vi "Get SubroutineInfo.vi"(11 "error in (no error)":errorcluster) -> (4 "data":T1, 15 "error out":errorcluster)   [LabVIEW 2021, in "Migrator Reusables.lvlib"]
uses:
  Migrator Reusables.lvlib
  controls/ErrorInformation.ctl
  controls/Dictionary States.ctl
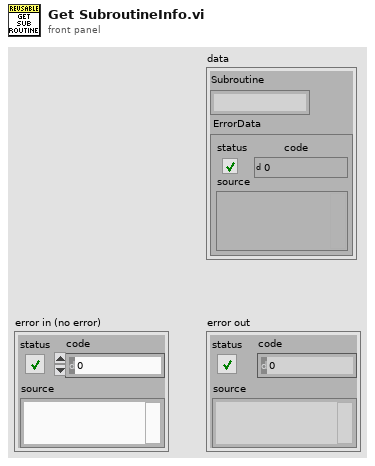
[diagram p1: front panel]
types:
  T1 = typedef "Migrator Reusables.lvlib/ErrorInformation.ctl" = cluster{"Subroutine":string, "ErrorData":errorcluster}
  T2 = typedef "Migrator Reusables.lvlib/Dictionary States.ctl" = enum16{"Set", "Get", "Delete", "Delete All"}
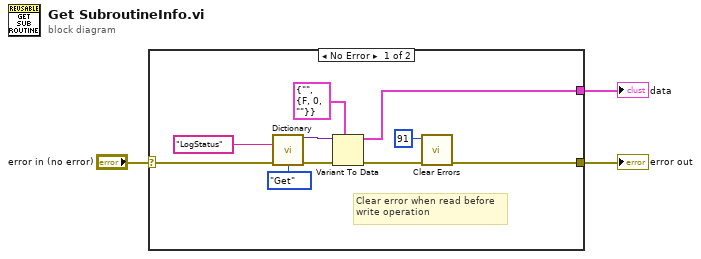
[diagram p0: block diagram]
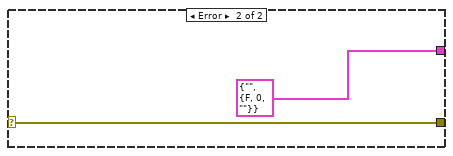
[diagram p2: hidden frame]
diagram:
  n1 = case shown="No Error" "error in (no error)" {
    selector: "error in (no error)" -> [w13 w15]
    tunnel: [w4 w15] -> w2
    tunnel: [w7 T1 {"Subroutine"="", "ErrorData"={"status"=FALSE, "code"=0, "source"=""}} ("ErrorInformation")] -> w1
    frame No Error {
      # "Clear error when read before\nwrite operation"
      n2 = call "Dictionary.vi"("Key"="LogStatus", "error in (no error)"=w13, "Dict States"=Dictionary_States."Get") -> ("Variant_Out"=w11:variant, "error out"=w12:errorcluster)  [unwired: 11 in]
      n3 = Variant To Data(error in=w12, type=T1 {"Subroutine"="", "ErrorData"={"status"=FALSE, "code"=0, "source"=""}} ("ErrorInformation"), Variant=w11) -> (data=w7:T1, error out=w6:errorcluster)
      n4 = call <vilib>:"Clear Errors.vi"("error in (no error)"=w6, "specific error code to clear (0: all)"=91) -> ("error out"=w4:errorcluster)  [unwired: 4 in, 1 out]
    }
    frame Error {
    }
  }
  "error out" <- w2
  "data" <- w1
